vi "Single Channel Strain Configure.vi"(5 "Channel":string, 6 "SampTime":dbl, 7 "SampCount":i32 format="%.0g", 8 "error in (no error)":errorcluster {"code" format="%.0x"}, 9 "GaugeFactor":dbl, 10 "GaugeResistance":dbl, 11 "instrument handle":refnum<k15>) -> (0 "error out":errorcluster {"code" format="%.0x"}, 3 "instrument handle out":refnum<k15>)   [LabVIEW 2020, in "Keysight DAQ970.lvlib"]
doc: "Configures a single channel for direct 2-wire strain gauge DMM digitizing, but they do not initiate the digitizing. This command redefines the scan list."
uses:
  Keysight DAQ970.lvlib
  KtDAQ970.dll
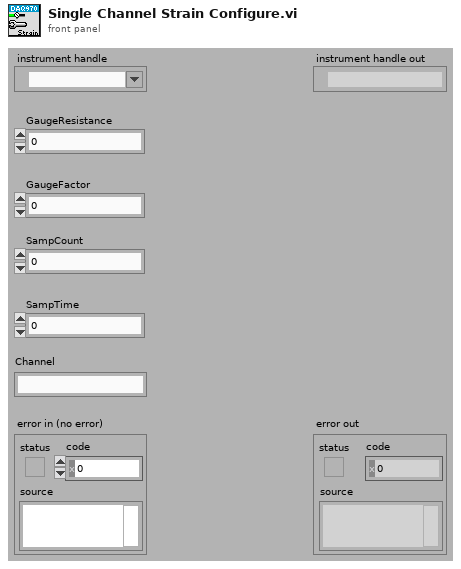
[diagram p1: front panel]
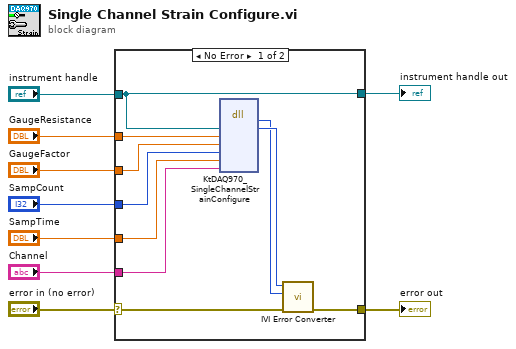
[diagram p0: block diagram]
diagram:
  n1 = case shown="No Error" "error in (no error)" {
    selector: "error in (no error)" -> [w17 w21]
    tunnel: [w16 w21] -> w9
    tunnel: "instrument handle" -> [w10 w20]
    tunnel: "GaugeResistance" -> [w15 _]
    tunnel: "GaugeFactor" -> [w14 _]
    tunnel: "SampCount" -> [w13 _]
    tunnel: "SampTime" -> [w12 _]
    tunnel: "Channel" -> [w11 _]
    tunnel: [w10 w20] -> w1
    frame No Error {
      n2 = dll-call lib="KtDAQ970**.dll" fn="KtDAQ970_SingleChannelStrainConfigure"("Vi"=w10, "GaugeResistance"=w15, "GaugeFactor"=w14, "SampCount"=w13, "SampTime"=w12, "Channel"=w11) -> (w18:i32, "Vi"=w19:u32)  [unwired: 8 in, 2 out]
      n3 = call "IVI Error Converter.vi"("error in (no error)"=w17, "IVI error code (0)"=w18, "instrument handle"=w19) -> ("error out"=w16:errorcluster)  [unwired: 7 in, 1 out]
    }
    frame Error {
    }
  }
  "error out" <- w9
  "instrument handle out" <- w1
